vi "fpga.sandbox.vi"   [LabVIEW 2022 SP3]
uses:
  orderbook/orderbook.state.ctl
types:
  T1 = typedef "orderbook.state.ctl" = enum16{"Reset", "WaitForNewCommand", "AddOrder", "Get.All.Orders", "Get.Top", "Order.Executed", "Reduce.Size", "Modify.Order", "Delete.Order"}
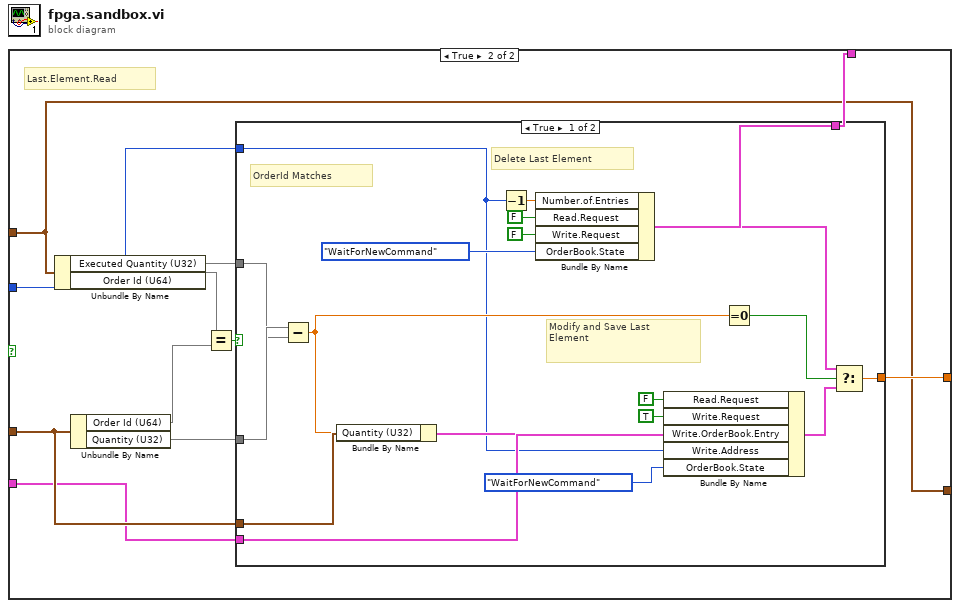
[diagram p0: block diagram]
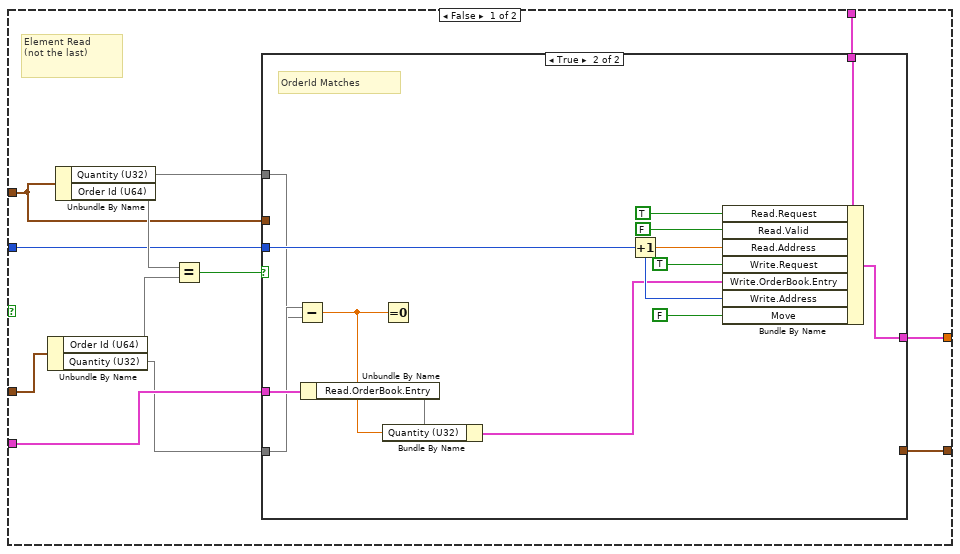
[diagram p2: hidden frame]
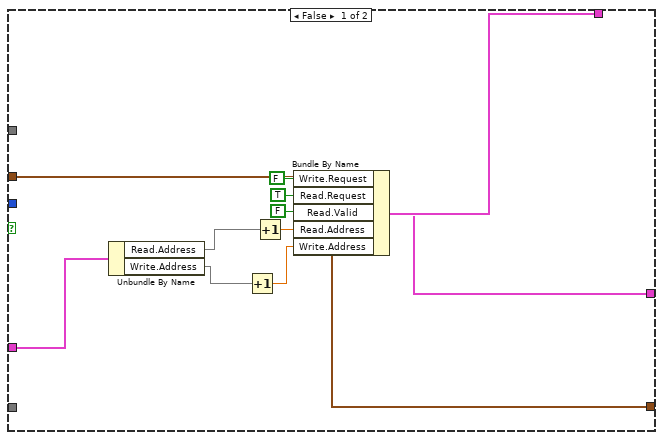
[diagram p3: hidden frame]
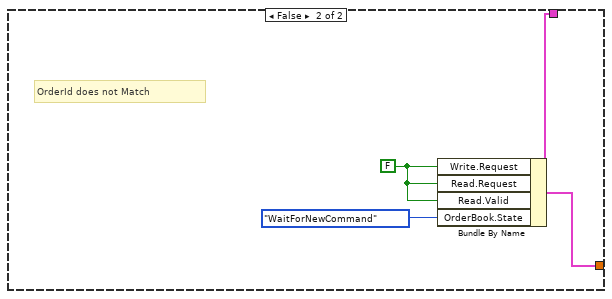
[diagram p4: hidden frame]
diagram:
  n1 = case shown="True" {
    selector: _ -> [_ _]
    tunnel: _ -> [w12 w48]
    tunnel: [w11 w47] -> _
    tunnel: _ -> [w8 w38]
    tunnel: _ -> [w5 w39]
    tunnel: _ -> [w9 w46]
    tunnel: [w7 w38] -> _
    tunnel: _ -> [w3 w40]
    frame False {
      # "Element Read\n(not the last)"
      n2 = Unbundle By Name(w3) -> ("Order Id (U64)"=w2, "Quantity (U32)"=w1)
      n3 = Unbundle By Name(w8) -> ("Quantity (U32)"=w6, "Order Id (U64)"=w10)
      n4 = Equal?(x=w10, y=w2) -> (x = y?=w4:bool)
      n5 = case shown="True" w4 {
        tunnel: w12 -> [w23 w37]
        tunnel: [w22 w36] -> w11
        tunnel: w9 -> [_ w35]
        tunnel: w8 -> [w17 _]
        tunnel: [w17 _] -> w7
        tunnel: w1 -> [_ w33]
        tunnel: w6 -> [_ w32]
        tunnel: w5 -> [w16 w34]
        frame False {
          n6 = Unbundle By Name(w16) -> ("Read.Address"=w15, "Write.Address"=w14)
          n7 = Increment(x=w14) -> (x+1=w13:dbl)
          n8 = Increment(x=w15) -> (x+1=w18:dbl)
          n9 = Bundle By Name(cluster=w23, "Write.Request"=FALSE, "Read.Request"=TRUE, "Read.Valid"=FALSE, "Read.Address"=w18, "Write.Address"=w13) -> (w22:cluster{})
        }
        frame True {
          # "OrderId Matches"
          n10 = Subtract(x=w33, y=w32) -> (x-y=w24:dbl)
          n11 = Unbundle By Name(w34) -> ("Read.OrderBook.Entry"=w25)
          n12 = Equal To 0?(x=w24) -> ()  [unwired: 1 out]
          n13 = Bundle By Name(cluster=w25, "Quantity (U32)"=w24) -> (w26:cluster{})
          n14 = Increment(x=w35) -> (x+1=w29:dbl)
          n15 = Bundle By Name(cluster=w37, "Read.Request"=TRUE, "Read.Valid"=FALSE, "Read.Address"=w29, "Write.Request"=TRUE, "Write.OrderBook.Entry"=w26, "Write.Address"=w35, "Move"=FALSE) -> (w36:cluster{})
        }
      }
    }
    frame True {
      # "Last.Element.Read"
      n16 = Unbundle By Name(w38) -> ("Executed Quantity (U32)"=w41, "Order Id (U64)"=w43)
      n17 = Unbundle By Name(w40) -> ("Order Id (U64)"=w45, "Quantity (U32)"=w42)
      n18 = Equal?(x=w43, y=w45) -> (x = y?=w44:bool)
      n19 = case shown="True" w44 {
        tunnel: w48 -> [w67 w71]
        tunnel: [w59 w70] -> w47
        tunnel: w46 -> [w49 _]
        tunnel: w40 -> [w57 _]
        tunnel: w42 -> [w62 _]
        tunnel: w41 -> [w61 _]
        tunnel: w39 -> [w55 _]
        frame True {
          # "Modify and Save Last\nElement"
          # "Delete Last Element"
          # "OrderId Matches"
          n20 = Subtract(x=w62, y=w61) -> (x-y=w56:dbl)
          n21 = Bundle By Name(cluster=w57, "Quantity (U32)"=w56) -> (w51:cluster{})
          n22 = Decrement(x=w49) -> (x-1=w64:dbl)
          n23 = Bundle By Name(cluster=w67, "Number.of.Entries"=w64, "Read.Request"=FALSE ("Write.Request"), "Write.Request"=FALSE ("Read.Request"), "OrderBook.State"=orderbook.state."WaitForNewCommand") -> (w58:cluster{})
          n24 = Bundle By Name(cluster=w55, "Read.Request"=FALSE ("Write.Request"), "Write.Request"=TRUE, "Write.OrderBook.Entry"=w51, "Write.Address"=w49, "OrderBook.State"=orderbook.state."WaitForNewCommand") -> (w54:cluster{})
          n25 = Equal To 0?(x=w56) -> (x = 0?=w60:bool)
          n26 = Select(t=w58, s=w60, f=w54) -> (s? t:f=w59:dbl)
        }
        frame False {
          w68 = FALSE ("Write.Request")
          # "OrderId does not Match"
          n27 = Bundle By Name(cluster=w71, "Write.Request"=w68, "Read.Request"=w68, "Read.Valid"=w68, "OrderBook.State"=orderbook.state."WaitForNewCommand") -> (w70:cluster{})
        }
      }
    }
  }
